vi "Analyze Temperature (broken Run button).vi"() -> ()   [LabVIEW 2019]
uses:
  <vilib>/DAQmx/create/channels.llb/DAQmx Create Channel (AI-Temperature-Thermocouple).vi
  <vilib>/DAQmx/read.llb/DAQmx Read (Analog DBL 1Chan 1Samp).vi
panel:
  out "In Range ?":string
  out "Current Temperature (deg F)":dbl
  out "Current Temperature (deg C)":dbl
  in  "Lower Limit (deg C)":dbl
  in  "Upper Limit (deg C)":dbl
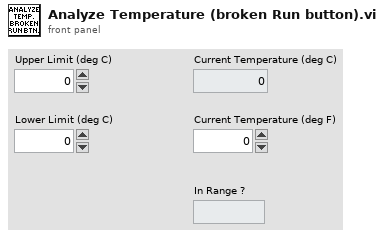
[diagram p1: front panel]
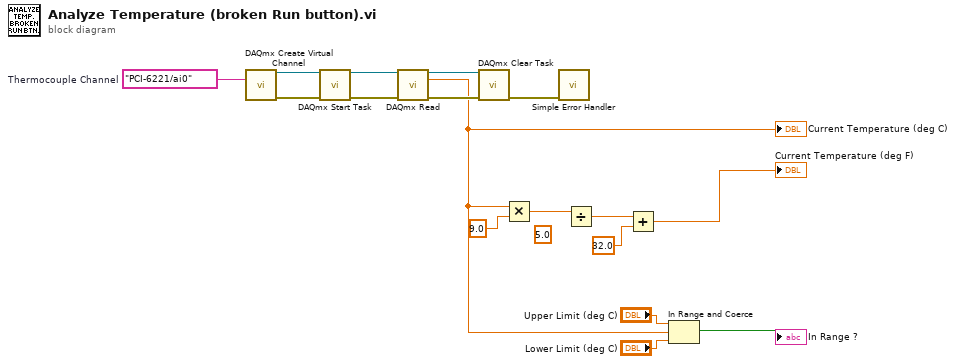
[diagram p0: block diagram]
diagram:
  (unwired) 5.0
  w17 = tag "PCI-6221/ai0"  # Thermocouple Channel
  n1 = call-poly <vilib>:"DAQmx Create Virtual Channel.vi"("physical channels"=w17) -> ("task out"=w16:refnum<k21>, "error out"=w15:errorcluster)  [unwired: 13 in]
  n2 = call <vilib>:"DAQmx Start Task.vi"("task/channels in"=w16, "error in"=w15) -> ("task out"=w14:refnum<k21>, "error out"=w13:errorcluster)  [unwired: 12 in]
  n3 = call-poly <vilib>:"DAQmx Read.vi"("task/channels in"=w14, "error in"=w13) -> ("task out"=w12:refnum<k21>, "data"=w3:dbl, "error out"=w11:errorcluster)  [unwired: 11 in]
  "Current Temperature (deg C)" <- w3
  n4 = call <vilib>:"DAQmx Clear Task.vi"("task in"=w12, "error in"=w11) -> ("error out"=w1:errorcluster)  [unwired: 13 in]
  n5 = Multiply(x=w3, y=9.0) -> (x*y=w9:dbl)
  n6 = call <vilib>:"Simple Error Handler.vi"("error in (no error)"=w1) -> ()  [unwired: 4 in, 5 out]
  n7 = Divide(x=w9) -> (x/y=w8:dbl)  [unwired: 1 in]
  n8 = Add(x=w8, y=32.0) -> (x+y=→"Current Temperature (deg F)":dbl)
  n9 = In Range and Coerce(upper limit="Upper Limit (deg C)", x=w3, lower limit="Lower Limit (deg C)") -> (In Range?=→"In Range ?":bool)  [unwired: 1 out]
